vi "hyst_sat_drift_cascade.vi"(4 "N_hyst":i32, 6 "N_sat":i32, 8 "Den":sgl[](array[numeric])=[0.982758, -1.98194, 1.0, 0.0, 0.0, 0.0, 0.0, 0.0, 0.0], 9 "Num":sgl[](array[numeric])=[-0.00254, 0.000408, 0.00295, 0.0, 0.0, 0.0, 0.0, 0.0, 0.0], 10 "TF Order":i32=2, 11 "u_k (un saturated)":fxp<+/-,32,5>) -> (2 "Hinv(uk)":fxp<+/-,32,10>)   [LabVIEW 2017]
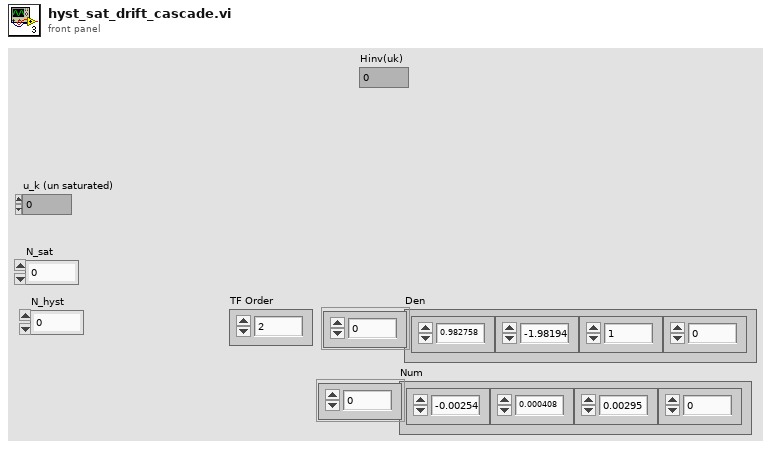
[diagram p1: front panel]
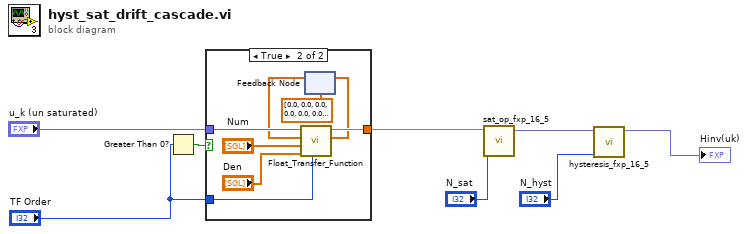
[diagram p0: block diagram]
diagram:
  n1 = Greater Than 0?(x="TF Order") -> (x > 0?=w4:bool)
  n2 = case shown="True" w4 {
    tunnel: "u_k (un saturated)" -> [w9 w17]
    tunnel: "TF Order" -> [_ w16]
    tunnel: [w9 w15] -> w2
    frame False {
    }
    frame True {
      n3 = feedback #1(sgl[] [0.0, 0.0, 0.0, 0.0, 0.0, 0.0, 0.0, 0.0, 0.0] ("State Out")) -> (w13:sgl[])
      n4 = call "Float_Transfer_Function.vi"("TF Order"=w16, "Den"="Den", "Num"="Num", "State In"=w13, "Input"=w17) -> ("State Out"=w14:sgl[], "Output"=w15:sgl)  [unwired: 4 in]
      n5 = feedback-in #1(w14) -> ()
    }
  }
  n6 = call "sat_op_fxp_16_5.vi"("N_sat"="N_sat", "uk_in"=w2) -> ("Hinv(uk)"=w8:fxp<+/-,32,10>)  [unwired: 9 in]
  n7 = call "hysteresis_fxp_16_5.vi"("N_hyst"="N_hyst", "uk_in"=w8) -> ("Hinv(uk)"=→"Hinv(uk)":fxp<+/-,32,10>)  [unwired: 9 in]
